vi "Configure Sample Clock Rate.vi"(8 "error in (no error)":errorcluster, 9 "Clock Rate (100 MHz)":dbl=100000000.0, 10 "Modulation Format (1: Dual Modulation)":u16(ring)=1 items=["Dual Modulation"=1, "Dual ARB"=2, "Multitone"=3, "Two-tone"=6, "AWGN ARB"=8], 11 "VISA resource name":refnum<visa-resource-name>) -> (0 "error out":errorcluster, 3 "VISA resource name out":refnum<visa-resource-name>)   [LabVIEW 2014, in "Agilent PSG MXG Series.lvlib"]
doc: "Configures the sample clock rate.\n\n<B>Notes:</B>\n(1) This VI is valid only in E8267C, E8257D, E8267D, N5162A, N5182A, N5172B, N5182B.\n\n(2) For E8267C, this VI is valid only when the instrument installs <B>Option 002</B> (Internal baseband generator) or <B>Option 602</B> (Digital bus baseband generator).\n\n(3) For E8267D, this VI is valid only when the instrument installs <B>Option 601</B> or <B>Option 602</B> (Internal baseband generator).\n\n(4) For N5162A and N5182A, this VI is valid only when the instrument installs <B>Option 651</B> or <B>Option 652</B> or <B>Option 654</B> (Internal baseband generator).\n\n(4) For N5172B and N5182B, this VI is valid only when the instrument installs <B>Option 431</B>."
uses:
  Agilent PSG MXG Series.lvlib
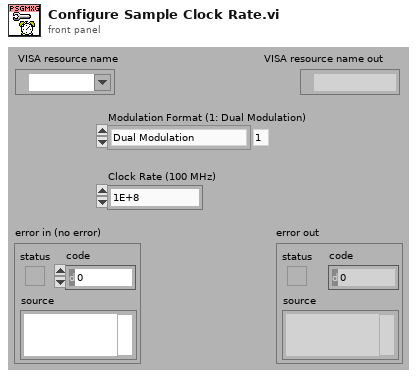
[diagram p1: front panel]
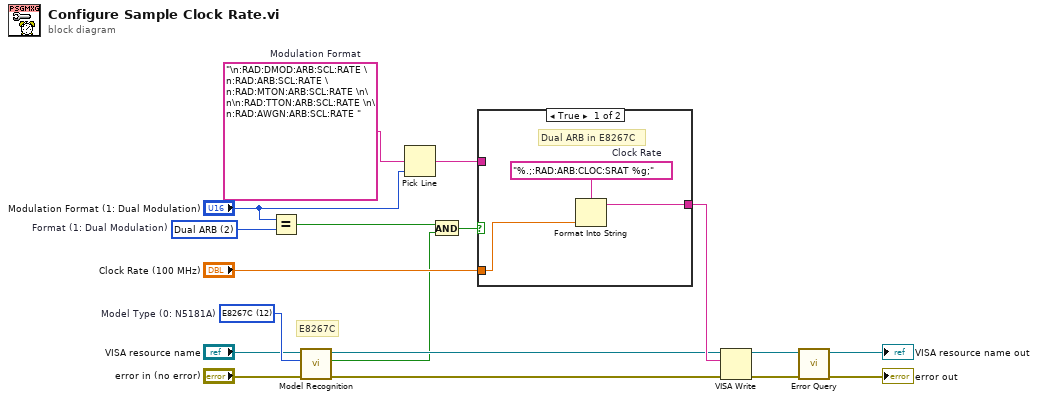
[diagram p0: block diagram]
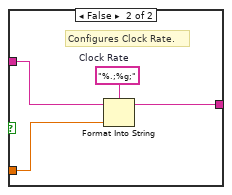
[diagram p2: hidden frame]
diagram:
  w8 = u16 12 items=["N5181A"=0, "N5182A"=1, "E8241A"=5, "E8244A"=6, "E8251A"=7, "E8254A"=8, "E8247C"=10, "E8257C"=11, "E8267C"=12, "E8257D"=15, "E8267D"=16]  # Model Type (0: N5181A)
  w11 = u16 2 items=["Dual Modulation"=1, "Dual ARB"=2]  # Format (1: Dual Modulation)
  w18 = "\n:RAD:DMOD:ARB:SCL:RATE \n:RAD:ARB:SCL:RATE \n:RAD:MTON:ARB:SCL:RATE \n\n\n:RAD:TTON:ARB:SCL:RATE \n\n:RAD:AWGN:ARB:SCL:RATE "  # Modulation Format
  # "E8267C"
  n1 = Equal?(x="Modulation Format (1: Dual Modulation)", y=w11) -> (x = y?=w9:bool)
  n2 = call "Model Recognition.vi"("error in (no error)"="error in (no error)", "Model Type (0: N5181A)"=w8, "VISA resource name"="VISA resource name") -> ("error out"=w7:errorcluster, "Is Model Correct"=w5:bool, "VISA resource name out"=w6:refnum<visa-resource-name>)  [unwired: 6 out]
  n3 = Pick Line(multi-line string=w18, line index="Modulation Format (1: Dual Modulation)") -> (output string=w17:string)  [unwired: 1 out]
  n4 = And(x=w9, y=w5) -> (x .and. y?=w10:bool)
  n5 = case shown="True" w10 {
    tunnel: w17 -> [_ w25]
    tunnel: "Clock Rate (100 MHz)" -> [w20 w23]
    tunnel: [w19 w22] -> w13
    frame True {
      w21 = "%.;:RAD:ARB:CLOC:SRAT %g;"  # Clock Rate
      # "Dual ARB in E8267C"
      n6 = Format Into String(format string=w21, w20) -> (resulting string=w19:string)  [unwired: 2 in, 1 out]
    }
    frame False {
      w24 = "%.;%g;"  # Clock Rate
      # "Configures Clock Rate."
      n7 = Format Into String(format string=w24, initial string=w25, w23) -> (resulting string=w22:string)  [unwired: 1 in, 1 out]
    }
  }
  n8 = VISA Write(VISA resource name=w6, write buffer=w13, error in (no error)=w7) -> (VISA resource name out=w15:refnum<visa-resource-name>, error out=w14:errorcluster)  [unwired: 1 out]
  n9 = call "Error Query.vi"("error in (no error)"=w14, "VISA resource name"=w15) -> ("error out"=→"error out":errorcluster, "VISA resource name out"=→"VISA resource name out":refnum<visa-resource-name>)  [unwired: 8 out]
